vi "Get single element.vi"(8 "error in (no error)":errorcluster, 9 "Variant in":variant, 11 "String":string) -> (0 "error out":errorcluster, 3 "Variant out":variant)   [LabVIEW 2015]
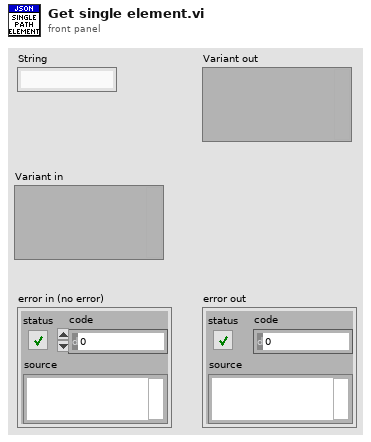
[diagram p1: front panel]
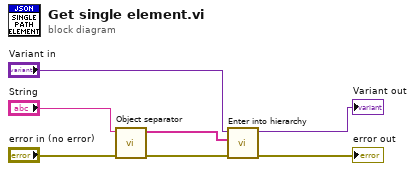
[diagram p0: block diagram]
diagram:
  n1 = call "Object separator.vi"("error in (no error)"="error in (no error)", "json path in"="String") -> ("error out"=w2:errorcluster, "output array of keys"=w5:string[])  [unwired: 8 in]
  n2 = call "Enter into hierarchy.vi"("error in (no error)"=w2, "output array of keys"=w5, "Variant in"="Variant in") -> ("error out"=→"error out":errorcluster, "Variant out"=→"Variant out":variant)  [unwired: 7 in]
